vi "Coordinate_transforms.vi"(1 "Traverse Name":string="EnFlo Tunnel", 2 "Input":sgl[](array[numeric])=[0.0, 0.0, 0.0] format="%.2f", 3 "Mode":enum16{"XYZ to Channel", "Channel to XYZ"}(ring)) -> (0 "Output":sgl[](array[numeric]) format="%.2f")   [LabVIEW 2022 SP3]
uses:
  DriveConfigGlobal.vi
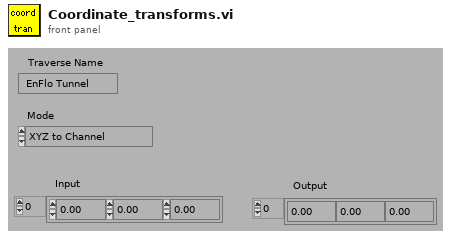
[diagram p1: front panel]
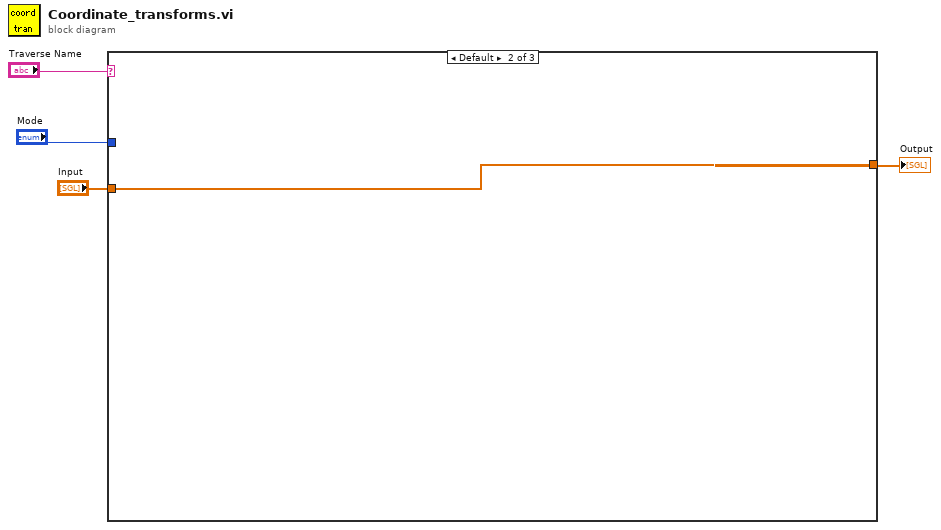
[diagram p0: block diagram]
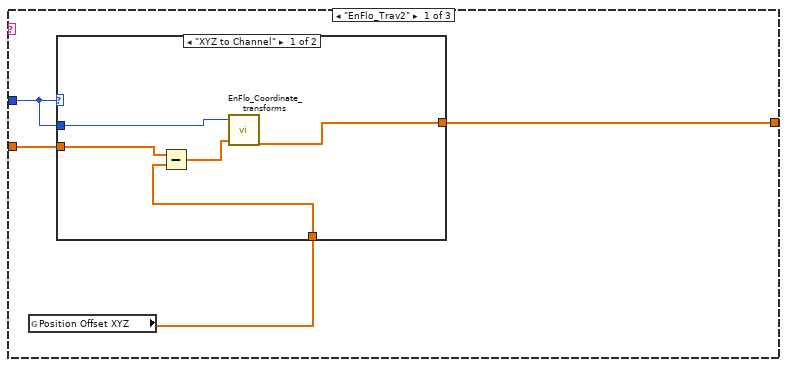
[diagram p2: hidden frame]
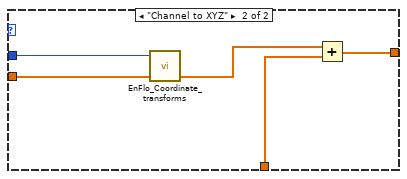
[diagram p3: hidden frame]
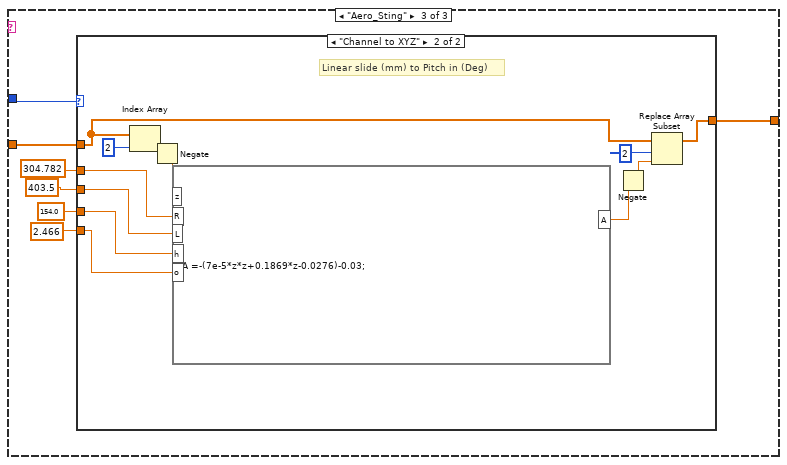
[diagram p4: hidden frame]
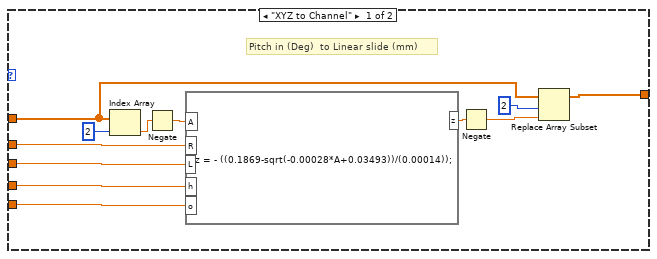
[diagram p5: hidden frame]
diagram:
  n1 = case shown="Default" "Traverse Name" {
    tunnel: "Input" -> [w8 w19 w25]
    tunnel: [w6 w19 w24] -> w3
    tunnel: "Mode" -> [w5 _ w26]
    frame "EnFlo_Trav2" {
      n2 = global read "DriveConfigGlobal.vi" "Position Offset XYZ"() -> (w7:dbl[])
      n3 = case shown="\"XYZ to Channel\"" w5 {
        tunnel: w8 -> [w11 w18]
        tunnel: w7 -> [w12 w16]
        tunnel: [w10 w15] -> w6
        tunnel: w5 -> [w9 w14]
        frame "XYZ to Channel" {
          n4 = Subtract(x=w11, y=w12) -> (x-y=w13:dbl[])
          n5 = call "EnFlo_Coordinate_transforms.vi"("Input"=w13, "Mode"=w9) -> ("Output"=w10:dbl[])  [unwired: 3 out]
        }
        frame "Channel to XYZ" {
          n6 = call "EnFlo_Coordinate_transforms.vi"("Input"=w18, "Mode"=w14) -> ("Output"=w17:dbl[])  [unwired: 3 out]
          n7 = Add(x=w17, y=w16) -> (x+y=w15:dbl[])
        }
      }
    }
    frame Default {
    }
    frame "Aero_Sting" {
      n8 = case shown="\"Channel to XYZ\"" w26 {
        tunnel: w25 -> [w37 w42]
        tunnel: [w29 w41] -> w24
        tunnel: 2.466 -> [w35 w49]
        tunnel: 304.782 -> [w34 w50]
        tunnel: 403.5 -> [w33 w47]
        tunnel: 154.0 -> [w32 w48]
        frame "XYZ to Channel" {
          # "Pitch in (Deg)  to Linear slide (mm)"
          n9 = Index Array(array=w37, index=2) -> (element=w31:sgl)
          n10 = Negate(x=w31) -> (-x=w28:sgl)
          n11 = formula code="z = - ((0.1869-sqrt(-0.00028*A+0.03493))/(0.00014));"("A"=w28, "R"=w34, "L"=w33, "h"=w32, "o"=w35) -> ("z"=w30:dbl)
          n12 = Negate(x=w30) -> (-x=w27:dbl)
          n13 = Replace Array Subset(array=w37, new element=w27, index=2) -> (w29:sgl[])
        }
        frame "Channel to XYZ" {
          # "Linear slide (mm) to Pitch in (Deg)"
          n14 = Index Array(array=w42, index=2) -> (element=w45:sgl)
          n15 = Negate(x=w45) -> (-x=w39:sgl)
          n16 = formula code="A =-(7e-5*z*z+0.1869*z-0.0276)-0.03;"("z"=w39, "R"=w50, "L"=w47, "h"=w48, "o"=w49) -> ("A"=w43:dbl)
          n17 = Negate(x=w43) -> (-x=w40:dbl)
          n18 = Replace Array Subset(array=w42, new element=w40, index=2) -> (w41:sgl[])
        }
      }
    }
  }
  "Output" <- w3
